vi "DSF.Engine.Framework.Increment Plugins.vi"(8 "error in (no error)":errorcluster, 11 "Framework in":refnum<class "DSF.Engine.Framework.lvclass">) -> (0 "error out":errorcluster, 3 "Framework out":refnum<class "DSF.Engine.Framework.lvclass">)   [LabVIEW 2017, in "DSF.Engine.lvlib" / "DSF.Engine.Framework.lvclass"]
uses:
  DSF.Engine.Framework.lvclass
  DSF.Engine.Framework.lvclass/DSF.Engine.Framework.ctl
  Plugin/DSF.Engine.Plugin.lvclass/DSF.Engine.Plugin.ctl
  Timing/DSF.Engine.Timing.lvclass/DSF.Engine.Timing.ctl
  Plugin/DSF.Engine.Plugin.Get Timing.vi
  Timing/DSF.Engine.Timing.Iteration.Increment.vi
  Plugin/DSF.Engine.Plugin.Set Timing.vi
  Timing/DSF.Engine.Timing.Is Active Cycle.vi
  Timing/DSF.Engine.Timing.Get Iteration.vi
  Timing/DSF.Engine.Timing.Set Iteration.vi
  Timing/DSF.Engine.Timing.Get Decimation.vi
  Timing/DSF.Engine.Timing.Get Offset.vi
  Plugin/DSF.Engine.Plugin.lvclass
  State/Framework State.lvclass
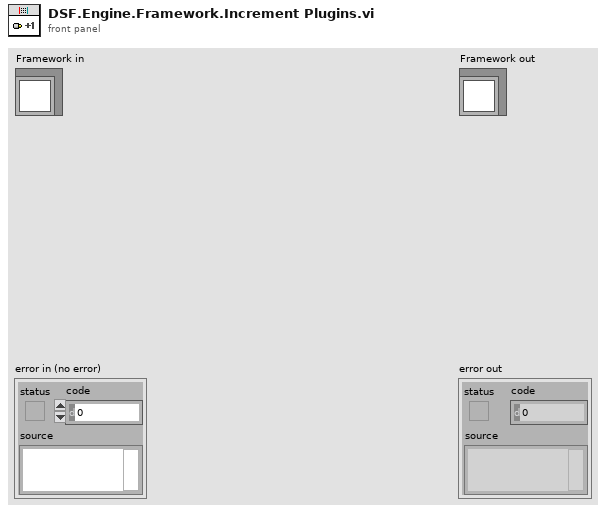
[diagram p1: front panel]
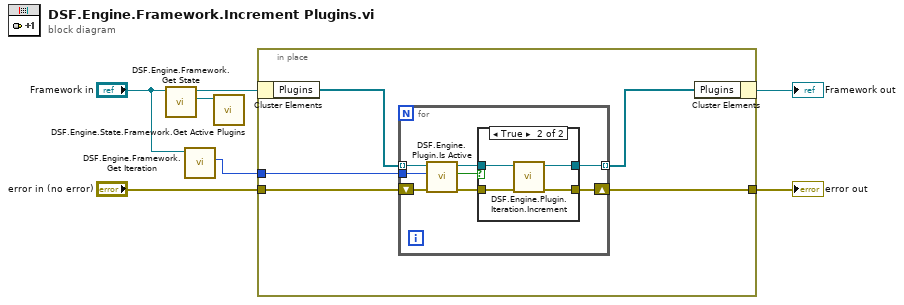
[diagram p0: block diagram]
diagram:
  n1 = call "DSF.Engine.Framework.Get State.vi"("Framework in"="Framework in") -> ("State"=w5:refnum<class "Framework State.lvclass">, "Framework out"=w2:refnum<class "DSF.Engine.Framework.lvclass">)  [unwired: 9 in]
  n2 = call "DSF.Engine.Framework.Get Iteration.vi"("Framework in"="Framework in") -> ("iteration"=w3:u64)  [unwired: 9 in, 1 out]
  n3 = call "DSF.Engine.State.Framework.Get Active Plugins.vi"("Framework State in"=w5) -> ()  [unwired: 9 in, 2 out]
  n4 = in-place {
    in-place-border: [w12] -> w7
    in-place-border: "error in (no error)" -> [w11]
    in-place-border: w3 -> [w10]
    n5 = in-place-cluster #1(w2) -> ("Plugins"=w9:refnum<class "DSF.Engine.Plugin.lvclass">[])
    n6 = for {
      tunnel: w9 -> [w16] mode=indexing
      tunnel: [w19] -> w8 mode=indexing
      shift-right: [w18] -> w12
      shift-left: w11 -> [w17]
      tunnel: w10 -> [w13]
      n7 = call "DSF.Engine.Plugin.Is Active.vi"("cycle count"=w13, "Plugin in"=w16) -> ("active this cycle?"=w14:bool, "Plugin out"=w15:refnum<class "DSF.Engine.Plugin.lvclass">)  [unwired: 8 in]
      n8 = case shown="True" w14 {
        tunnel: [w20 w25] -> w19
        tunnel: [w21 w24] -> w18
        tunnel: w17 -> [w21 w23]
        tunnel: w15 -> [w20 w22]
        frame False {
        }
        frame True {
          n9 = call "DSF.Engine.Plugin.Iteration.Increment.vi"("error in (no error)"=w23, "Plugin in"=w22) -> ("error out"=w24:errorcluster, "Plugin out"=w25:refnum<class "DSF.Engine.Plugin.lvclass">)  [unwired: 8 in]
        }
      }
    }
    n10 = in-place-cluster #1("Plugins"=w8) -> (→"Framework out":refnum<class "DSF.Engine.Framework.lvclass">)
  }
  "error out" <- w7
